vi "Periodic Tasks.vi"(8 "error in":errorcluster) -> ()   [LabVIEW 2013]
doc: "This VI runs in parallel to other tasks. It can contain as many user-defined periodic loops as you need. These can carry out PID or other sorts of timed response."
uses:
  <vilib>/Rock Robotics/SystemInterfaces/Utilities/FPGA_UtilitiesLED Source.ctl
  <vilib>/Rock Robotics/SystemInterfaces/Utilities/FPGA_UtilitiesLED State.ctl
  Robot Global Data.vi
  <vilib>/Rock Robotics/WPI/Joystick/WPI_JoystickGetSetRefNum.vi
panel:
  in  "Throw Motor Speed (-1 to 1)":dbl(slide)=-1.0 min=-1.0 max=1.0 step=0.05 scale=-1.0..1.0 scale format="%#.3f"
  out "Throw Motor Running":bool
  out "Throw Joystick State":bool
  out "Throw Switch State":bool
  out "Lift Motor Speed":dbl
  in  "Lift Motor Speed Up":dbl(slide)=0.49999999999999994 min=-1.0 max=1.0 step=0.05 scale=0.0..1.0 scale format="%#.3f"
  in  "Lift Motor Speed Down":dbl(slide)=0.25 min=-1.0 max=1.0 step=0.05 scale=0.0..1.0 scale format="%#.3f"
  out "Lift Motor Running":bool
  out "Joystick Lift State":bool
  out "Lift Motor Direction":bool
  out "Lift Switch B State":bool
  out "Lift Switch A State":bool
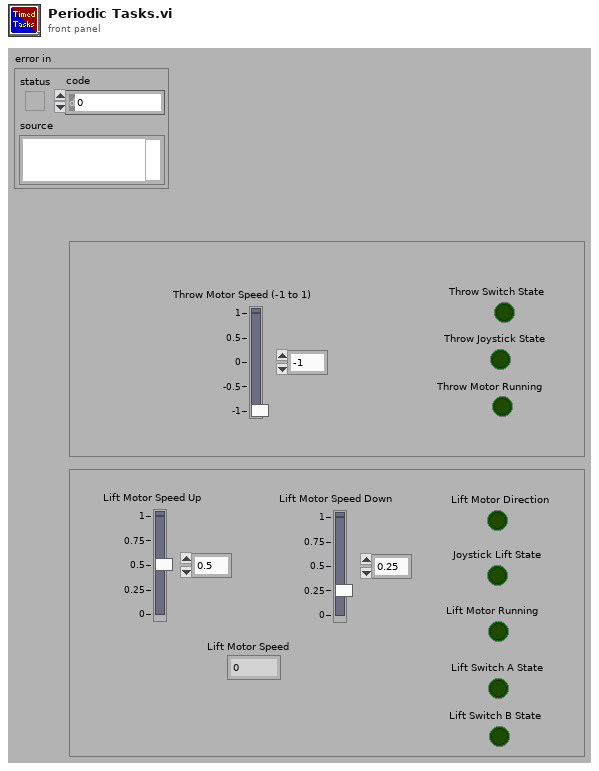
[diagram p1: front panel]
types:
  T1 = typedef "WPI_MotorControlDeviceRef.ctl" = cluster{"DeviceStatus":errorcluster, "Type":enum16{"PWM", "CAN"}, "PWM":cluster{"Digital Module":T2, "PWM Channel":T3, "DeadBand":T4}, "CAN":cluster{"Device Number":u8, "Control Mode":T5, "Semaphore":T6, "Max Vout":dbl}, "Invert":bool, "TransformRef":T7, "InvTransformRef":T7}
  T2 = typedef "FPGA_TypedefDigitalModule.ctl" = enum16{"Digital Module 1", "Digital Module 2"}
  T3 = typedef "FPGA_DIOPWMChannel.ctl" = enum8{"PWM 1", "PWM 2", "PWM 3", "PWM 4", "PWM 5", "PWM 6", "PWM 7", "PWM 8", "PWM 9", "PWM 10", "Invalid"}
  T4 = typedef "WPI_PWMDeadband.ctl" = cluster{"Name":string, "maxPositivePwm":i32, "minPositivePwm":i32, "centerPwm":i32, "maxNegativePwm":i32, "minNegativePwm":i32, "angularRange":u16}
  T5 = typedef "WPI_CANJaguar_ControlMode.ctl" = enum8{"Percent VBus", "Current", "Speed", "Position", "Voltage"}
  T6 = typedef "Semaphore RefNum" = refnum<k1>
  T7 = typedef "WPI_PWMTransform_ConPane.ctl" = refnum<vi>
  T8 = typedef "WPI_JoystickDevRef.ctl" = cluster{"Device":T9}
  T9 = typedef "WPI_JoystickDeviceEnum.ctl" = enum16{"USB 1", "USB 2", "USB 3", "USB 4", "Kinect 1", "Kinect 2"}
  T10 = cluster{"MotorControlDevRef":T1, "JoystickDevRef":T8}
  T11 = cluster{"JoystickDevRef":T8, "MotorControlDevRef":T1}
  T12 = typedef "WPI_DigitalInputDevRef.ctl" = cluster{"DevStatus":errorcluster, "DIO Channel":T13, "Digital Module":T2}
  T13 = typedef "FPGA_DIOChannel.ctl" = enum8{"DIO 1", "DIO 2", "DIO 3", "DIO 4", "DIO 5", "DIO 6", "DIO 7", "DIO 8", "DIO 9", "DIO 10", "DIO 11", "DIO 12", "DIO 13", "DIO 14", "Invalid"}
  T14 = typedef "FPGA_UtilitiesLED State.ctl" = enum16{"Off", "On", "Toggle"}
  T15 = typedef "FPGA_UtilitiesLED Source.ctl" = enum16{"User LED", "FPGA LED"}
  T16 = typedef "WPI_JoystickButtonState.ctl" = cluster{"Button 1":bool, "Button 2":bool, "Button 3":bool, "Button 4":bool, "Button 5":bool, "Button 6":bool, "Button 7":bool, "Button 8":bool, "Button 9":bool, "Button 10":bool, "Button 11":bool, "Button 12":bool}
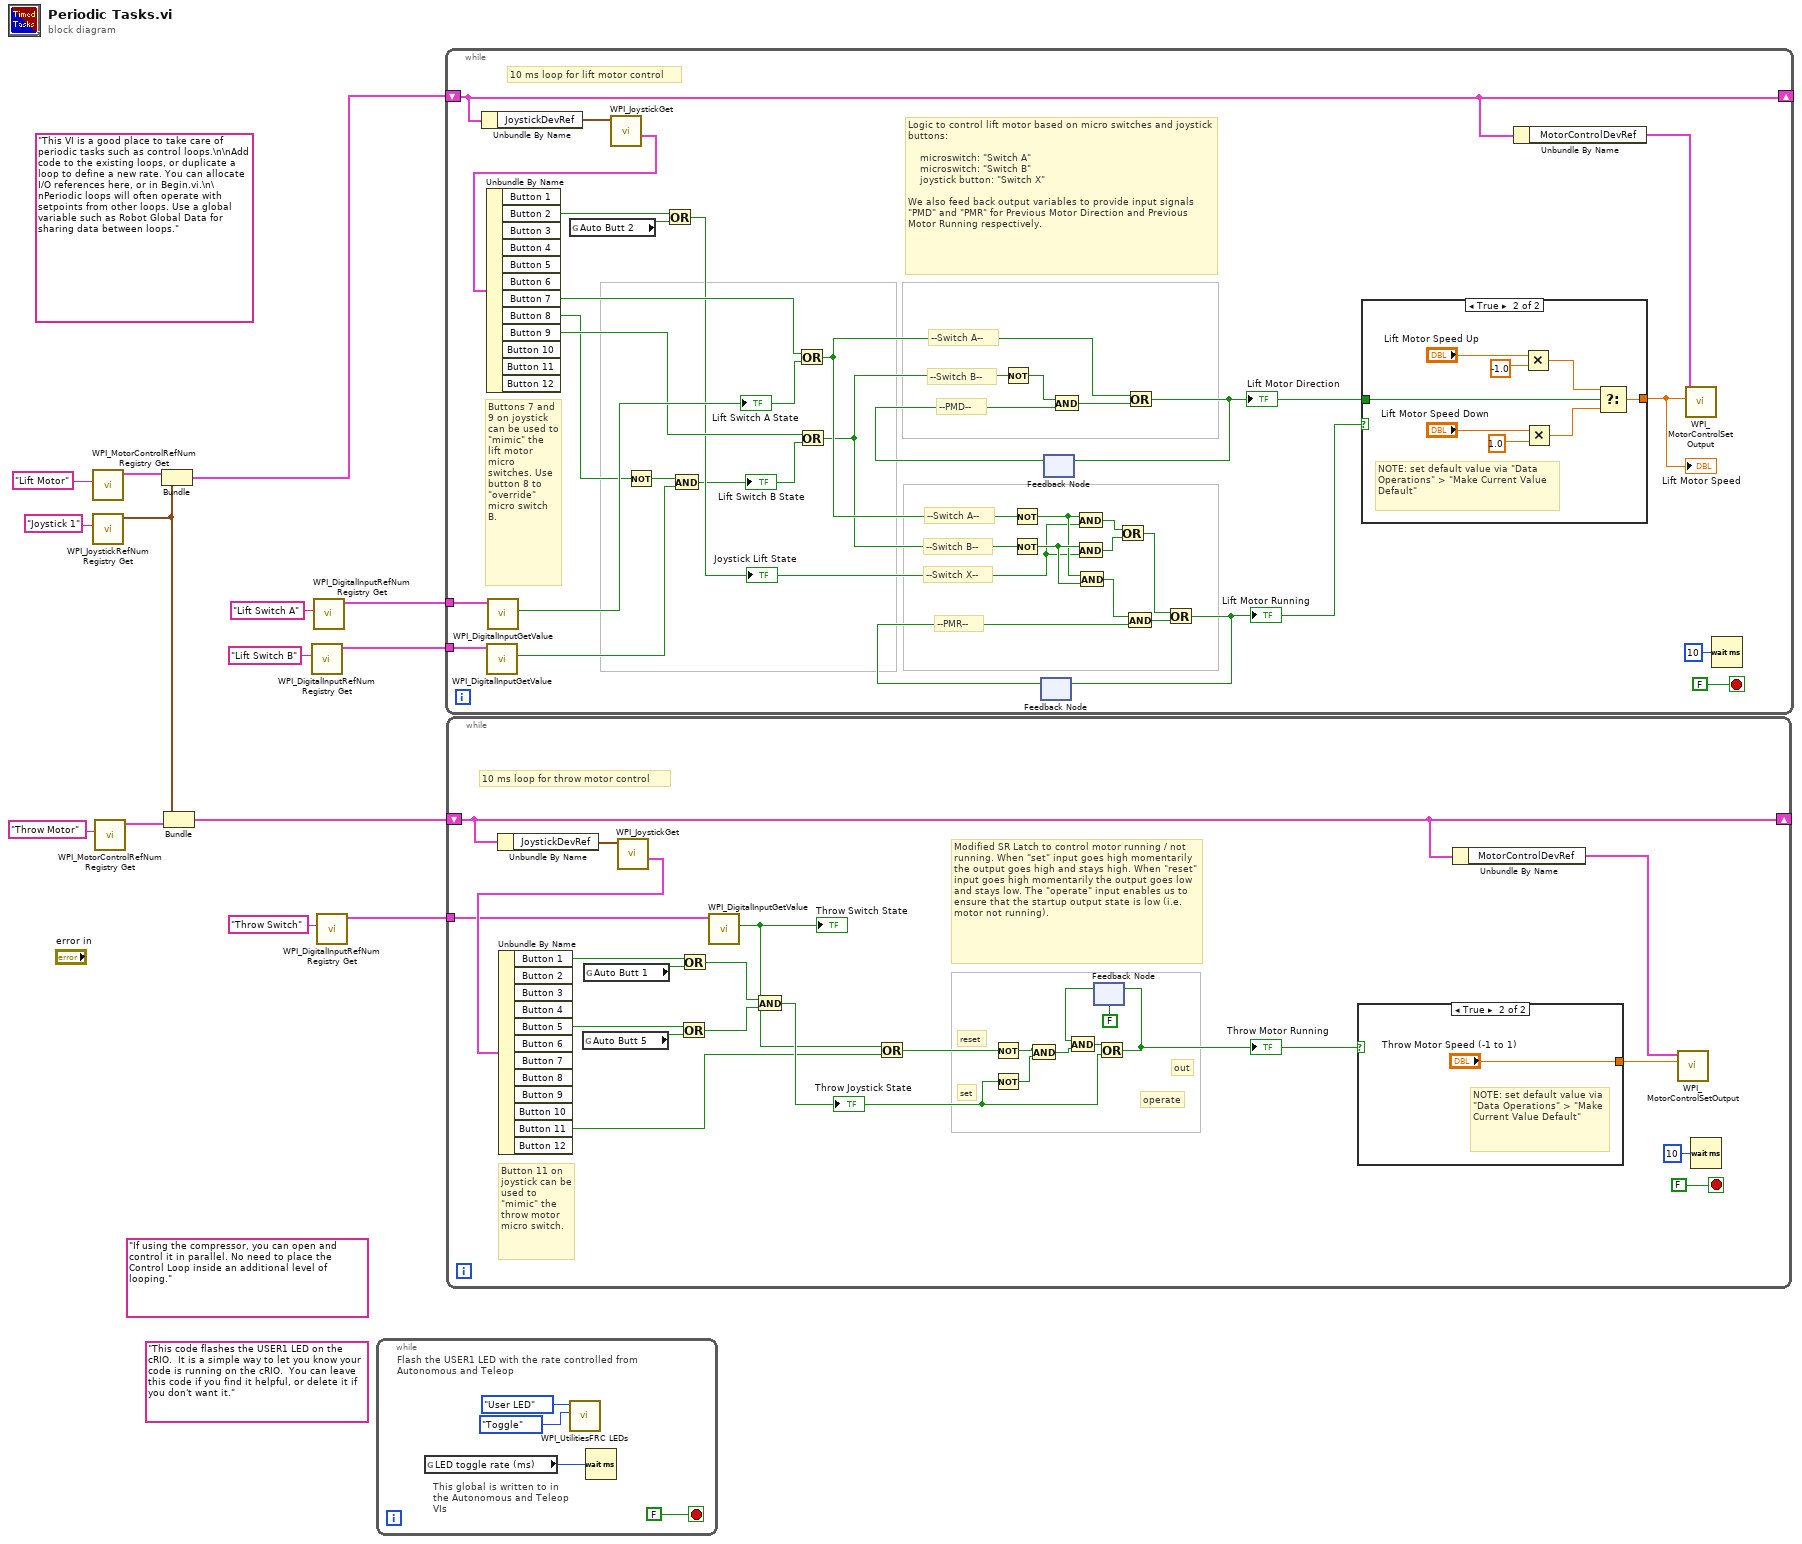
[diagram p0: block diagram]
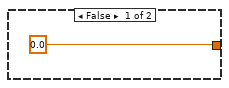
[diagram p2: hidden frame]
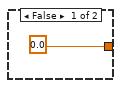
[diagram p3: hidden frame]
diagram:
  (unwired) "If using the compressor, you can open and control it in parallel. No need to place the Control Loop inside an additional level of looping."
  (unwired) "This code flashes the USER1 LED on the cRIO.  It is a simple way to let you know your code is running on the cRIO.  You can leave this code if you find it helpful, or delete it if you don't want it."
  (unwired) "This VI is a good place to take care of periodic tasks such as control loops.\n\nAdd code to the existing loops, or duplicate a loop to define a new rate. You can allocate I/O references here, or in Begin.vi.\n\nPeriodic loops will often operate with setpoints from other loops. Use a global variable such as Robot Global Data for sharing data between loops."
  n1 = call <vilib>:"WPI_MotorControlRefNum Registry Get.vi"("refnum name"="Lift Motor") -> ("MotorControlDevRef"=w6:T1)  [unwired: 9 in, 1 out]
  n2 = call <vilib>:"WPI_JoystickRefNum Registry Get.vi"("refnum name"="Joystick 1") -> ("JoystickDevRef"=w5:T8)  [unwired: 1 in, 9 out]
  n3 = call <vilib>:"WPI_MotorControlRefNum Registry Get.vi"("refnum name"="Throw Motor") -> ("MotorControlDevRef"=w11:T1)  [unwired: 9 in, 1 out]
  n4 = Bundle("MotorControlDevRef"=w6, "JoystickDevRef"=w5) -> (w13:T10)  [unwired: 1 out]
  n5 = Bundle("JoystickDevRef"=w5, "MotorControlDevRef"=w11) -> (w10:T11)  [unwired: 1 in]
  n6 = call <vilib>:"WPI_DigitalInputRefNum Registry Get.vi"("refnum name"="Lift Switch B") -> ("DigitalInputDevRef"=w2:T12)  [unwired: 9 in, 1 out]
  n7 = call <vilib>:"WPI_DigitalInputRefNum Registry Get.vi"("refnum name"="Lift Switch A") -> ("DigitalInputDevRef"=w3:T12)  [unwired: 9 in, 1 out]
  n8 = call <vilib>:"WPI_DigitalInputRefNum Registry Get.vi"("refnum name"="Throw Switch") -> ("DigitalInputDevRef"=w1:T12)  [unwired: 9 in, 1 out]
  n9 = while {
    stop <- FALSE stop-if-true
    # "This global is written to in the Autonomous and Teleop VIs"
    # "Flash the USER1 LED with the rate controlled from Autonomous and Teleop"
    n10 = global read "Robot Global Data.vi" "LED toggle rate (ms)"() -> (w15:u32)
    n11 = call <vilib>:"WPI_UtilitiesFRC LEDs.vi"("State"=FPGA_UtilitiesLED_State."Toggle", "LED Type"=FPGA_UtilitiesLED_Source."User LED") -> ()  [unwired: 1 in, 9 out]
    n12 = Wait (ms)(milliseconds to wait=w15) -> ()  [unwired: 1 out]
  }
  n13 = while {
    shift-right: [w33] -> _
    shift-left: w13 -> [w33]
    tunnel: w3 -> [w32]
    tunnel: w2 -> [w31]
    stop <- FALSE stop-if-true
    # "Buttons 7 and 9 on joystick can be used to \"mimic\" the lift motor micro switches. Use button 8 to \"override\" micro switch B."
    # "Logic to control lift motor based on micro switches and joystick buttons:\n\n    microswitch: \"Switch A\"\n    microswitch: \"Switch B\"\n    joystick button: \"Switch X\"\n\nWe also feed back output variables to provide input signals \"PMD\" and \"PMR\" for Previous Motor Direction and Previous Motor Running respectively."
    # "--PMR--"
    # "--Switch X--"
    # "--Switch B--"
    # "--Switch A--"
    # "--PMD--"
    # "--Switch B--"
    # "--Switch A--"
    # "10 ms loop for lift motor control"
    n14 = Unbundle By Name(w33) -> ("JoystickDevRef"=w36:T8)
    n15 = call <vilib>:"WPI_DigitalInputGetValue.vi"("DigitalInputDevRef"=w31) -> ("Value"=w22:bool)  [unwired: 8 in, 2 out]
    n16 = call <vilib>:"WPI_DigitalInputGetValue.vi"("DigitalInputDevRef"=w32) -> ("Value"=w28:bool)  [unwired: 8 in, 2 out]
    "Lift Switch A State" <- w28
    n17 = global read "Robot Global Data.vi" "Auto Butt 2"() -> (w25:bool)
    n18 = call <vilib>:"WPI_JoystickGet.vi"("JoystickDevRef"=w36) -> ("Buttons"=w35:T16)  [unwired: 4 in, 2 out]
    n19 = Unbundle By Name(w35) -> ("Button 2"=w23:bool, "Button 7"=w29:bool, "Button 8"=w20:bool, "Button 9"=w26:bool)  [unwired: 8 out]
    n20 = Not(x=w20) -> (.not. x?=w19:bool)
    n21 = Or(x=w23, y=w25) -> (x .or. y?=w24:bool)
    "Joystick Lift State" <- w24
    n22 = And(x=w19, y=w22) -> (x .and. y?=w21:bool)
    "Lift Switch B State" <- w21
    n23 = Or(x=w29, y=w28) -> (x .or. y?=w30:bool)
    n24 = Or(x=w26, y=w21) -> (x .or. y?=w27:bool)
    n25 = Not(x=w27) -> (.not. x?=w37:bool)
    n26 = Not(x=w30) -> (.not. x?=w45:bool)
    n27 = Not(x=w27) -> (.not. x?=w46:bool)
    n28 = feedback #1() -> (w48:bool)  [unwired: 1 in]
    n29 = feedback #2() -> (w39:bool)  [unwired: 1 in]
    n30 = And(x=w37, y=w39) -> (x .and. y?=w38:bool)
    n31 = And(x=w45, y=w24) -> (x .and. y?=w42:bool)
    n32 = And(x=w46, y=w24) -> (x .and. y?=w41:bool)
    n33 = And(x=w45, y=w46) -> (x .and. y?=w47:bool)
    n34 = Or(x=w42, y=w41) -> (x .or. y?=w43:bool)
    n35 = And(x=w47, y=w48) -> (x .and. y?=w44:bool)
    n36 = Or(x=w30, y=w38) -> (x .or. y?=w40:bool)
    "Lift Motor Direction" <- w40
    n37 = feedback-in #2(w40) -> ()
    n38 = Or(x=w43, y=w44) -> (x .or. y?=w49:bool)
    "Lift Motor Running" <- w49
    n39 = feedback-in #1(w49) -> ()
    n40 = case shown="True" w49 {
      tunnel: w40 -> [_ w61]
      tunnel: [0.0 ("Throw Motor Speed (-1 to 1) 2") w55] -> w50
      frame False {
      }
      frame True {
        # "NOTE: set default value via \"Data Operations\" > \"Make Current Value Default\""
        n41 = Multiply(x="Lift Motor Speed Up", y=-1.0) -> (x*y=w59:dbl)
        n42 = Multiply(x="Lift Motor Speed Down", y=1.0) -> (x*y=w56:dbl)
        n43 = Select(t=w59, s=w61, f=w56) -> (s? t:f=w55:dbl)
      }
    }
    "Lift Motor Speed" <- w50
    n44 = Unbundle By Name(w33) -> ("MotorControlDevRef"=w34:T1)
    n45 = call <vilib>:"WPI_MotorControlSetOutput.vi"("Output"=w50, "MotorControlDevRef"=w34) -> ()  [unwired: 3 in, 7 out]
    n46 = Wait (ms)(milliseconds to wait=u32 10) -> ()  [unwired: 1 out]
  }
  n47 = while {
    shift-right: [w72] -> _
    shift-left: w10 -> [w72]
    tunnel: w1 -> [w71]
    stop <- FALSE stop-if-true
    # "Button 11 on joystick can be used to \"mimic\" the throw motor micro switch."
    # "Modified SR Latch to control motor running / not running. When \"set\" input goes high momentarily the output goes high and stays high. When \"reset\" input goes high momentarily the output goes low and stays low. The \"operate\" input enables us to ensure that the startup output state is low (i.e. motor not running)."
    # "operate"
    # "out"
    # "reset"
    # "set"
    # "10 ms loop for throw motor control"
    n48 = Unbundle By Name(w72) -> ("JoystickDevRef"=w75:T8)
    n49 = global read "Robot Global Data.vi" "Auto Butt 5"() -> (w63:bool)
    n50 = global read "Robot Global Data.vi" "Auto Butt 1"() -> (w67:bool)
    n51 = call <vilib>:"WPI_JoystickGet.vi"("JoystickDevRef"=w75) -> ("Buttons"=w74:T16)  [unwired: 4 in, 2 out]
    n52 = Unbundle By Name(w74) -> ("Button 1"=w66:bool, "Button 5"=w64:bool, "Button 11"=w68:bool)  [unwired: 9 out]
    n53 = Or(x=w64, y=w63) -> (x .or. y?=w62:bool)
    n54 = Or(x=w66, y=w67) -> (x .or. y?=w65:bool)
    n55 = call <vilib>:"WPI_DigitalInputGetValue.vi"("DigitalInputDevRef"=w71) -> ("Value"=w69:bool)  [unwired: 8 in, 2 out]
    "Throw Switch State" <- w69
    n56 = And(x=w65, y=w62) -> (x .and. y?=w82:bool)
    "Throw Joystick State" <- w82
    n57 = Or(x=w69, y=w68) -> (x .or. y?=w70:bool)
    n58 = Not(x=w70) -> (.not. x?=w76:bool)
    n59 = Not(x=w82) -> (.not. x?=w77:bool)
    n60 = And(x=w76, y=w77) -> (x .and. y?=w79:bool)
    n61 = feedback #3(FALSE) -> (w80:bool)
    n62 = And(x=w80, y=w79) -> (x .and. y?=w78:bool)
    n63 = Or(x=w78, y=w82) -> (x .or. y?=w84:bool)
    "Throw Motor Running" <- w84
    n64 = feedback-in #3(w84) -> ()
    n65 = case shown="True" w84 {
      tunnel: [0.0 ("Throw Motor Speed (-1 to 1) 2") "Throw Motor Speed (-1 to 1)"] -> w81
      frame False {
      }
      frame True {
        # "NOTE: set default value via \"Data Operations\" > \"Make Current Value Default\""
      }
    }
    n66 = Unbundle By Name(w72) -> ("MotorControlDevRef"=w73:T1)
    n67 = call <vilib>:"WPI_MotorControlSetOutput.vi"("Output"=w81, "MotorControlDevRef"=w73) -> ()  [unwired: 3 in, 7 out]
    n68 = Wait (ms)(milliseconds to wait=u32 10) -> ()  [unwired: 1 out]
  }
